vi "FGV_TDMS.vi"(7 "GET/SET":T1, 11 "Prop in":T2) -> (3 "Prop out":T2)   [LabVIEW 2021]
uses:
  Typedefs/FGV_TDMS.ctl
  Typedefs/GET_SET.ctl
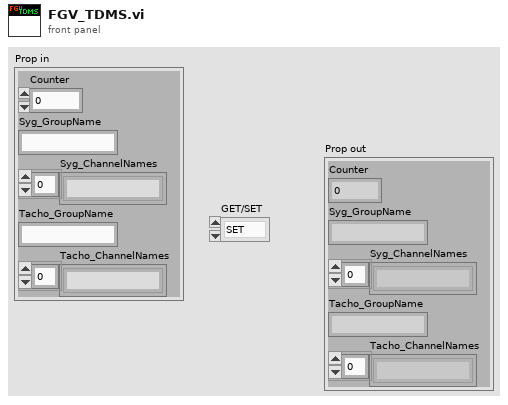
[diagram p1: front panel]
types:
  T1 = typedef "GET_SET.ctl" = enum16{"SET", "GET"}
  T2 = typedef "FGV_TDMS.ctl" = cluster{"Counter":i32, "Syg_GroupName":string, "Syg_ChannelNames":string[], "Tacho_GroupName":string, "Tacho_ChannelNames":string[]}
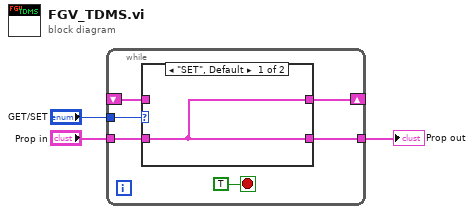
[diagram p0: block diagram]
diagram:
  n1 = while {
    tunnel: "GET/SET" -> [w9]
    shift-right: [w4] -> _
    shift-left: _ -> [w7]
    tunnel: "Prop in" -> [w6]
    tunnel: [w5] -> w1
    stop <- TRUE stop-if-true
    n2 = case shown="\"SET\", Default" w9 {
      tunnel: w7 -> [_ w11]
      tunnel: w6 -> [w10 _]
      tunnel: [w10 w11] -> w5
      tunnel: [w10 w11] -> w4
      frame "SET", Default {
      }
      frame "GET" {
      }
    }
  }
  "Prop out" <- w1
